vi "FreqC.Read Message.vi"(8 "error in (no error)":errorcluster, 10 "timeout in ms (-1)":i32, 11 "FreqC Message Session in":T2) -> (0 "error out":errorcluster, 1 "type":T1, 2 "data":dbl, 3 "FreqC Message Session out":T2)   [LabVIEW 2018]
uses:
  typedefs/FreqC.Message Session.ctl
  typedefs/FreqC.Message.ctl
  typedefs/FreqC.Message Type.ctl
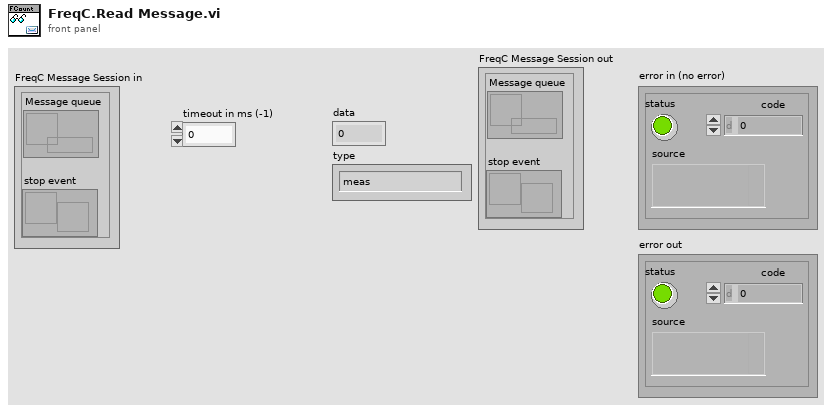
[diagram p1: front panel]
types:
  T1 = typedef "FreqC.Message Type.ctl" = enum16{"meas", "set level", "set gate"}
  T2 = typedef "FreqC.Message Session.ctl" = cluster{"Message queue":refnum<queue>, "stop event":refnum<user-event>}
  T3 = typedef "FreqC.Message.ctl" = cluster{"Message type":T1, "data":dbl}
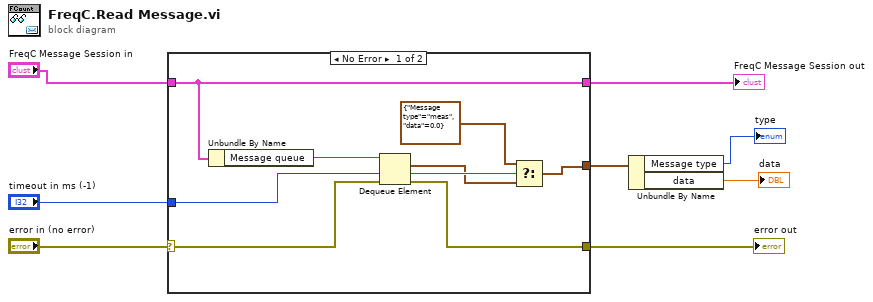
[diagram p0: block diagram]
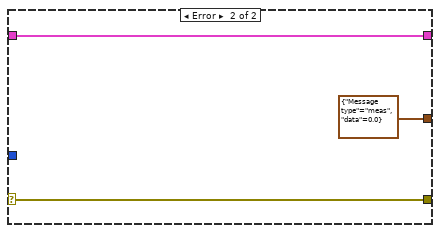
[diagram p2: hidden frame]
diagram:
  n1 = case shown="No Error" "error in (no error)" {
    selector: "error in (no error)" -> [w15 w20]
    tunnel: "FreqC Message Session in" -> [w17 w19]
    tunnel: [w17 w19] -> w1
    tunnel: [w14 w20] -> w2
    tunnel: "timeout in ms (-1)" -> [w13 _]
    tunnel: [w10 T3 {"Message type"=enum."meas", "data"=0.0} ("FreqC.Message")] -> w5
    frame No Error {
      n2 = Unbundle By Name(w17) -> ("Message queue"=w16:refnum<queue>)
      n3 = Dequeue Element(queue=w16, timeout in ms (-1)=w13, error in (no error)=w15) -> (element=w11:T3, timed out?=w12:bool, error out=w14:errorcluster)  [unwired: 1 out]
      n4 = Select(t=T3 {"Message type"=enum."meas", "data"=0.0}, s=w12, f=w11) -> (s? t:f=w10:T3)
    }
    frame Error {
    }
  }
  "FreqC Message Session out" <- w1
  "error out" <- w2
  n5 = Unbundle By Name(w5) -> ("Message type"=→"type":T1, "data"=→"data":dbl)
